vi "pico_move.vi"(9 "?":bool, 10 "Velocity":dbl(slide) scale=-10.0..10.0, 11 "Motor #":i32=1) -> ()   [LabVIEW 2013]
panel:
  out "ID List":string[](array[string])
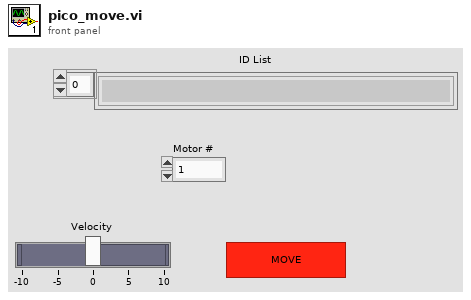
[diagram p1: front panel]
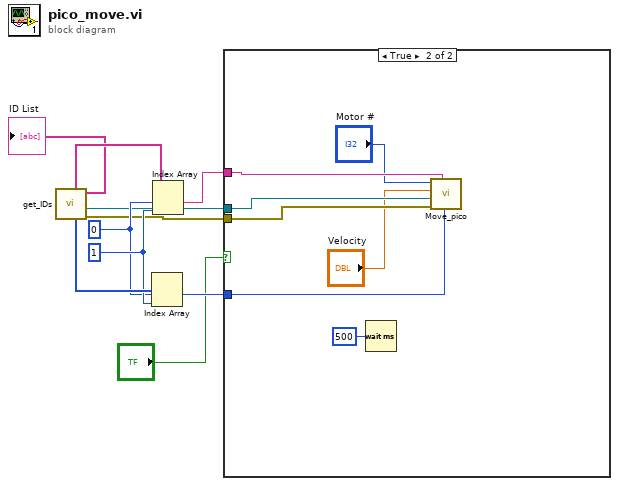
[diagram p0: block diagram]
diagram:
  w7 = 1 ("index")
  w6 = 0 ("index")
  n1 = call "get_IDs.vi"() -> ("error out 3"=w3:errorcluster, "CmdLib Out"=w2:refnum<k24>, "Identification List"=→"ID List":string[], "IDs"=w8:i32[], "Device Key"=w10:string[])  [unwired: 6 in, 1 out]
  n2 = Index Array(array=w8, index #1=w6, index #2=w7) -> (element #1=w5:i32)  [unwired: 1 out]
  n3 = Index Array(array=w10, index #1=w6, index #2=w7) -> (element #1=w4:string)  [unwired: 1 out]
  n4 = case shown="True" "?" {
    tunnel: w5 -> [_ w17]
    tunnel: w4 -> [_ w16]
    tunnel: w3 -> [_ w15]
    tunnel: w2 -> [_ w14]
    frame False {
    }
    frame True {
      n5 = Wait (ms)(milliseconds to wait=u32 500) -> ()  [unwired: 1 out]
      n6 = call "Move_pico.vi"("Device Address In"=w17, "DeviceKey In"=w16, "error in (no error)"=w15, "CmdLib In"=w14, "Relative Steps"="Velocity", "Motor #"="Motor #") -> ()  [unwired: 4 in, 2 out]
    }
  }
